vi "Percent Encode - OAuth.vi"(1 "unescaped string in":string) -> (0 "escaped string out":string)   [LabVIEW 2011, in "i3-oauth.lvlib"]
doc: "Percent encodes the supplied string."
uses:
  i3-oauth.lvlib
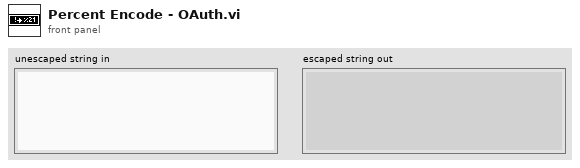
[diagram p1: front panel]
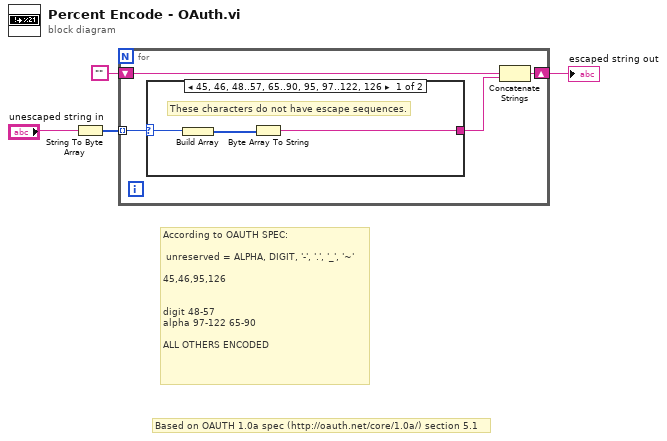
[diagram p0: block diagram]
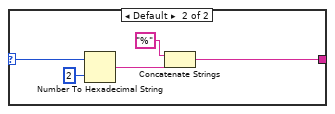
[diagram p2: hidden frame]
diagram:
  # "Based on OAUTH 1.0a spec (http://oauth.net/core/1.0a/) section 5.1"
  # "According to OAUTH SPEC:\n\n unreserved = ALPHA, DIGIT, '-', '.', '_', '~'\n\n45,46,95,126\n\n\ndigit 48-57\nalpha 97-122 65-90\n\nALL OTHERS ENCODED"
  n1 = String To Byte Array(string="unescaped string in") -> (unsigned byte array=w1:u8[])
  n2 = for {
    shift-right: [w5] -> w4
    shift-left: "" -> [w6]
    tunnel: w1 -> [w8] mode=indexing
    n3 = case shown="45, 46, 48..57, 65..90, 95, 97..122, 126" w8 {
      selector: w8 -> [w11 w14]
      tunnel: [w9 w13] -> w7
      frame 45, 46, 48..57, 65..90, 95, 97..122, 126 {
        # "These characters do not have escape sequences."
        n4 = Build Array(w11) -> (w10:u8[])
        n5 = Byte Array To String(unsigned byte array=w10) -> (string=w9:string)
      }
      frame Default {
        n6 = Number To Hexadecimal String(1:i16 2 ("width (-)"), 2:w14) -> (0:w15:string)
        n7 = Concatenate Strings("%" ("string"), w15) -> (w13:string)
      }
    }
    n8 = Concatenate Strings(w6, w7) -> (w5:string)
  }
  "escaped string out" <- w4
